vi "Output Range and Manual Status.vi"(8 "error in (no error)":errorcluster, 10 "Output (1:1)":u16(ring)=1 items=["1"=1, "2"=2, "3"=3, "4"=4], 11 "VISA resource name":refnum<visa-resource-name>) -> (0 "error out":errorcluster, 1 "Manual Output (0.00 %)":dbl format="%.2f", 2 "Range (0:Off)":u16(ring) items=["Off", "Low (On)", "Medium", "High"], 3 "VISA resource name out":refnum<visa-resource-name>)   [LabVIEW 2013, in "Lake Shore 336.lvlib"]
doc: "This VI returns the Range and Manual Output Value for the Heater Outputs and the Unpowered Analog Outputs."
uses:
  Lake Shore 336.lvlib
  Instance           1 38Saved   Output Range and Manual Status .vi
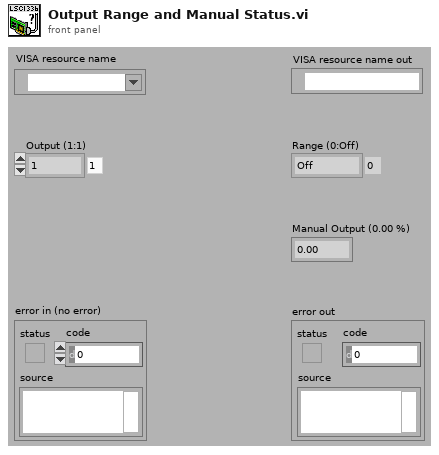
[diagram p1: front panel]
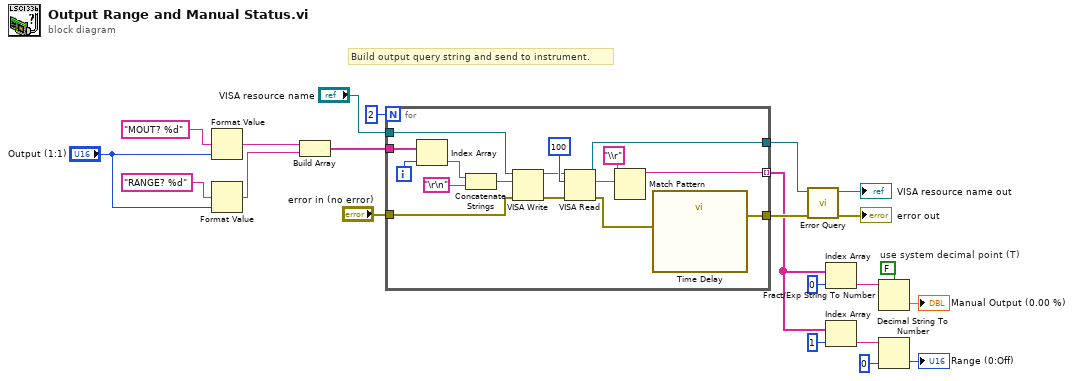
[diagram p0: block diagram]
diagram:
  w22 = FALSE  # use system decimal point (T)
  # "Build output query string and send to instrument."
  n1 = Format Value(format string="MOUT? %d", value (0)="Output (1:1)") -> (output string=w3:string)  [unwired: 1 in]
  n2 = Format Value(format string="RANGE? %d", value (0)="Output (1:1)") -> (output string=w2:string)  [unwired: 1 in]
  n3 = Build Array(w3, w2) -> (w15:string[])
  n4 = for {
    N: 2 -> [_]
    tunnel: [w32] -> w21
    tunnel: [w26] -> w20
    tunnel: "VISA resource name" -> [w31]
    tunnel: "error in (no error)" -> [w30]
    tunnel: w15 -> [w29]
    tunnel: [w28] -> w10 mode=indexing
    i -> [w33]
    n5 = Index Array(array=w29, index=w33) -> (element=w24:string)
    n6 = Concatenate Strings(w24, "\r\n") -> (w25:string)
    n7 = VISA Write(VISA resource name=w31, write buffer=w25, error in (no error)=w30) -> (VISA resource name out=w35:refnum<visa-resource-name>, error out=w34:errorcluster)  [unwired: 1 out]
    n8 = VISA Read(VISA resource name=w35, byte count=100, error in (no error)=w34) -> (VISA resource name out=w32:refnum<visa-resource-name>, read buffer=w37:string, error out=w27:errorcluster)  [unwired: 1 out]
    n9 = Match Pattern(string=w37, regular expression="\\r") -> (before substring=w28:string)  [unwired: 1 in, 3 out]
    n10 = call "Time Delay"("error in (no error)"=w27) -> ("error out"=w26:errorcluster)  [unwired: 10 in]
  }
  n11 = call "Error Query.vi"("error in (no error)"=w20, "VISA resource name"=w21) -> ("error out"=→"error out":errorcluster, "VISA resource name out"=→"VISA resource name out":refnum<visa-resource-name>)  [unwired: 7 in, 1 out]
  n12 = Index Array(array=w10, index=0) -> (element=w8:string)
  n13 = Index Array(array=w10, index=1) -> (element=w9:string)
  n14 = Fract/Exp String To Number(use system decimal point (T)=w22, string=w8) -> (number=→"Manual Output (0.00 %)":dbl)  [unwired: 2 in, 1 out]
  n15 = Decimal String To Number(string=w9, default (0L)=u16 0) -> (number=→"Range (0:Off)":u16)  [unwired: 1 in, 1 out]
